vi "Get Value Variant.vi"(8 "error in (no error)":errorcluster, 10 "value":variant, 11 "value pointer in":i64) -> (0 "error out":errorcluster, 2 "value out":variant, 3 "value pointer out":i64)   [LabVIEW 2020, in "Value.lvlib"]
uses:
  Value.lvlib
  3e63842f-1b42-44b7-bfbc-53574ae558bd.vi
  94649a53-8ca4-4095-9f16-4726c07ca332.vi
  0df52538-0c37-4fc1-a2a6-aa64d23bd73e.vi
  d57c28cb-9096-4c65-b10b-a5dea6344eea.vi
  ea7cb730-9445-4e63-a674-7488b051f0a2.vi
  a983453c-48a8-483e-9635-4b6015360bbf.vi
  ecc6d044-d1d6-4258-b554-93b542f000c4.vi
  3184ba56-7df3-4453-b731-c59013ebea68.vi
  f0dd0353-13dc-4229-be36-72f5216b3ba3.vi
  6054442b-7a6b-42bc-83b9-383781339b04.vi
  663b7534-5be4-4c26-8693-775dffd107bf.vi
  6affac03-527b-4ec4-b0fc-9a513264455a.vi
  6d95b702-a3d4-47fa-b99c-6e9c691d9abd.vi
  a9131e02-a07e-4dd8-b605-98a98183cd4d.vi
  334379f0-c2c1-4fd4-b37a-a75153a3c3c1.vi
  df721e5c-d840-4c3d-88a1-754951405b27.vi
  22215a59-2fe5-468e-8a76-07a567f1422d.vi
  37bd5290-b6b7-48eb-a0fa-e2d498b26fe2.vi
  3b673ad6-c2bb-415d-ac32-dac8d0585a62.vi
  1f354738-e960-4e7d-8bfb-2b975031cf57.vi
  4907590c-51dd-452d-854a-3f23d6337043.vi
  eb45627c-0224-4171-a2ca-7d038fcf7cb5.vi
  91e94b60-106e-4a8f-bb72-5d9817169e6a.vi
  763b9c78-21ee-42ab-85a7-a612ad3e0854.vi
  c7390ac7-e1e0-4f30-b90a-9159575d946d.vi
  b475763c-3eeb-44d5-9789-6e92f77c8c05.vi
  aaf6655d-cd8e-45f8-b77e-a22837ed21e0.vi
  7e13b756-e5dd-4f30-8145-3e48ab5751a0.vi
  830d96f2-0dcb-4e12-99cb-9e6dde05f73e.vi
  311b836b-25cf-44d6-867a-da423852ab29.vi
  77dc8c9c-6059-4e17-8748-14fb7ec0ac2f.vi
  884a57a7-1cc5-4241-a283-3421418f3c32.vi
  a9875d30-4bd9-4a8c-a52c-f68dec12aa6b.vi
  e5b34253-12a8-4f36-ae48-ef8a9a19dc9f.vi
  6dbc08b8-92b8-4054-99f1-d97896c52856.vi
  9a6462e7-f1a7-4896-b94c-43e163632ccd.vi
  c55a9e90-05cb-4a8a-8098-6274f5663967.vi
  919939b4-f74b-49d6-a078-a721f5adc92b.vi
  316c9c8d-b543-4ebf-942d-59175514938d.vi
  7b5734c8-9551-4087-a43c-2e9c6be36d77.vi
  229b0493-3b28-4ef3-8240-f1556a969e00.vi
  e7c0ed72-c8d2-4a6e-8d95-57b650344be6.vi
  76e9d66a-8186-463b-a0b5-702645c41f9e.vi
  78a636ab-c8c7-43d5-9c2f-ed25fd418a22.vi
  c324c6c0-264f-44f1-9003-e2f03347ce10.vi
  3f976d8e-f489-4d6c-8102-c644feb36fb3.vi
  99229403-bf4d-41b1-8e34-2119cf99b534.vi
  2b071918-53f3-414b-a359-069b1376627a.vi
  <vilib>/Utility/error.llb/Clear Errors.vi
  <vilib>/Utility/Data Type/Get Type Information.vi
  <vilib>/Utility/Data Type/Get Array Information.vi
  <vilib>/Utility/error.llb/Error Cluster From Error Code.vi
  Get Library Path.vi
  <vilib>/ErrorRing/Error Ring.xnode
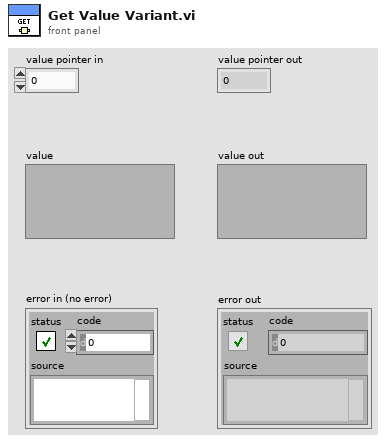
[diagram p1: front panel]
types:
  T1 = typedef "Value.lvlib/TypeCode.ctl" = enum8{"Null", "Bool", "BoolA", "Int8", "Int8A", "Int16", "Int16A", "Int32", "Int32A", "Int64", "Int64A", "UInt8", "UInt8A", "UInt16", "UInt16A", "UInt32", "UInt32A", "UInt64", "UInt64A", "Float32", "Float32A", "Float64", "Float64A", "String", "StringA", "Struct", "StructA", "Union", "UnionA", "Any", "AnyA"}
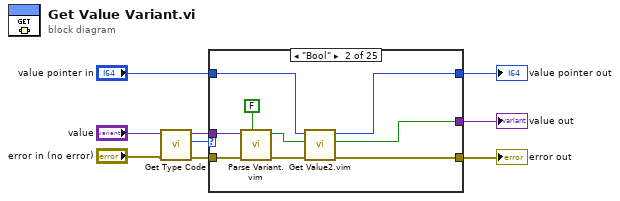
[diagram p0: block diagram]
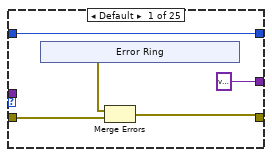
[diagram p2: hidden frame]
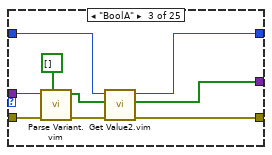
[diagram p3: hidden frame]
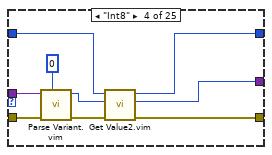
[diagram p4: hidden frame]
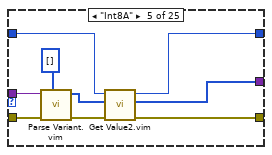
[diagram p5: hidden frame]
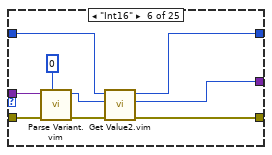
[diagram p6: hidden frame]
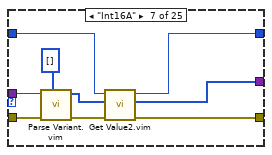
[diagram p7: hidden frame]
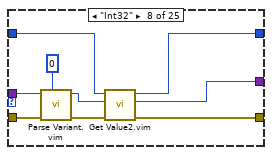
[diagram p8: hidden frame]
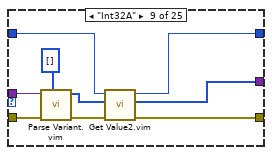
[diagram p9: hidden frame]
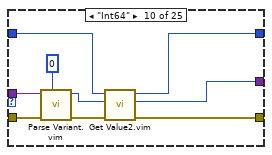
[diagram p10: hidden frame]
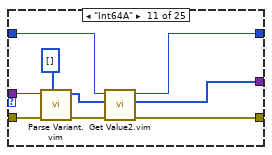
[diagram p11: hidden frame]
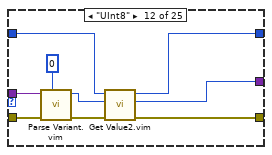
[diagram p12: hidden frame]
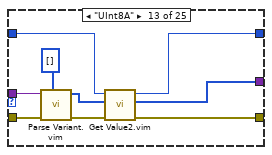
[diagram p13: hidden frame]
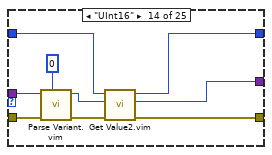
[diagram p14: hidden frame]
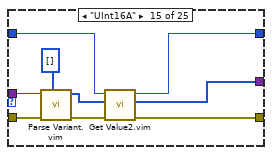
[diagram p15: hidden frame]
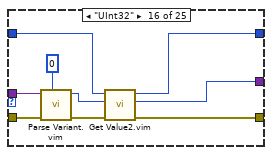
[diagram p16: hidden frame]
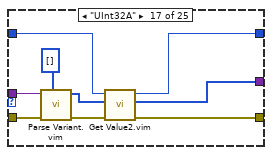
[diagram p17: hidden frame]
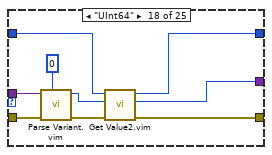
[diagram p18: hidden frame]
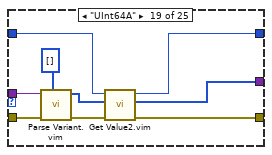
[diagram p19: hidden frame]
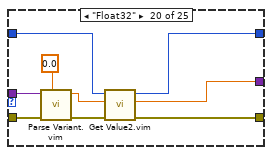
[diagram p20: hidden frame]
diagram:
  n1 = call "Get Type Code.vi"("error in (no error)"="error in (no error)", "value"="value") -> ("error out"=w7:errorcluster, "type code"=w6:T1, "value dup"=w5:variant)  [unwired: 5 in]
  n2 = case shown="\"Bool\"" w6 {
    tunnel: [w13 w24 w34 w43 w52 w61 w70 w79 w88 w97 w107 w115 w124 w133 w142 w151 w160 w169 w178 w187 w196 w205 w214 w223 w232] -> w1
    tunnel: w7 -> [w14 w27 w36 w45 w54 w63 w72 w81 w90 w99 w108 w117 w126 w135 w144 w153 w162 w171 w180 w189 w198 w207 w216 w225 w234]
    tunnel: [w10 w22 w32 w42 w50 w59 w68 w77 w86 w95 w105 w113 w122 w132 w140 w149 w159 w167 w176 w185 w194 w203 w212 w221 w230] -> w3
    tunnel: w5 -> [_ w21 w31 w41 w49 w58 w67 w76 w85 w94 w104 w112 w121 w131 w139 w148 w158 w166 w175 w184 w193 w202 w211 w220 w229]
    tunnel: [variant w20 w29 w39 w47 w56 w65 w74 w83 w92 w102 w110 w119 w129 w137 w146 w156 w164 w173 w182 w191 w200 w209 w218 w227] -> w2
    tunnel: "value pointer in" -> [w10 w19 w28 w38 w46 w55 w64 w73 w82 w91 w100 w109 w118 w128 w136 w145 w155 w163 w172 w181 w190 w199 w208 w217 w226]
    frame Default {
      n3 = xnode "Error Ring"() -> ("error out"=w12:errorcluster)
      n4 = Merge Errors(w12, w14) -> (w13:errorcluster)
    }
    frame "Bool" {
      n5 = call "Parse Variant.vim"("default"=FALSE, "error in (no error)"=w27, "value"=w21) -> ("error out"=w25:errorcluster, "value out"=w23:bool)  [unwired: 7 in]
      n6 = call "Get Value2.vim"("error in"=w25, "default"=w23, "value pointer in"=w19) -> ("error out"=w24:errorcluster, "value"=w20:bool, "value pointer out"=w22:i64)  [unwired: 6 in]
    }
    frame "BoolA" {
      n7 = call "Parse Variant.vim"("default"=bool[] [], "error in (no error)"=w36, "value"=w31) -> ("error out"=w35:errorcluster, "value out"=w33:bool[])  [unwired: 7 in]
      n8 = call "Get Value2.vim"("error in"=w35, "default"=w33, "value pointer in"=w28) -> ("error out"=w34:errorcluster, "value"=w29:bool[], "value pointer out"=w32:i64)  [unwired: 6 in]
    }
    frame "Int8" {
      n9 = call "Parse Variant.vim"("default"=i8 0, "error in (no error)"=w45, "value"=w41) -> ("error out"=w44:errorcluster, "value out"=w37:i8)  [unwired: 7 in]
      n10 = call "Get Value2.vim"("error in"=w44, "default"=w37, "value pointer in"=w38) -> ("error out"=w43:errorcluster, "value"=w39:i8, "value pointer out"=w42:i64)  [unwired: 6 in]
    }
    frame "Int8A" {
      n11 = call "Parse Variant.vim"("default"=i8[] [], "error in (no error)"=w54, "value"=w49) -> ("error out"=w53:errorcluster, "value out"=w51:i8[])  [unwired: 7 in]
      n12 = call "Get Value2.vim"("error in"=w53, "default"=w51, "value pointer in"=w46) -> ("error out"=w52:errorcluster, "value"=w47:i8[], "value pointer out"=w50:i64)  [unwired: 6 in]
    }
    frame "Int16" {
      n13 = call "Parse Variant.vim"("default"=i16 0, "error in (no error)"=w63, "value"=w58) -> ("error out"=w62:errorcluster, "value out"=w60:i16)  [unwired: 7 in]
      n14 = call "Get Value2.vim"("error in"=w62, "default"=w60, "value pointer in"=w55) -> ("error out"=w61:errorcluster, "value"=w56:i16, "value pointer out"=w59:i64)  [unwired: 6 in]
    }
    frame "Int16A" {
      n15 = call "Parse Variant.vim"("default"=i16[] [], "error in (no error)"=w72, "value"=w67) -> ("error out"=w71:errorcluster, "value out"=w69:i16[])  [unwired: 7 in]
      n16 = call "Get Value2.vim"("error in"=w71, "default"=w69, "value pointer in"=w64) -> ("error out"=w70:errorcluster, "value"=w65:i16[], "value pointer out"=w68:i64)  [unwired: 6 in]
    }
    frame "Int32" {
      n17 = call "Parse Variant.vim"("default"=0, "error in (no error)"=w81, "value"=w76) -> ("error out"=w80:errorcluster, "value out"=w78:i32)  [unwired: 7 in]
      n18 = call "Get Value2.vim"("error in"=w80, "default"=w78, "value pointer in"=w73) -> ("error out"=w79:errorcluster, "value"=w74:i32, "value pointer out"=w77:i64)  [unwired: 6 in]
    }
    frame "Int32A" {
      n19 = call "Parse Variant.vim"("default"=i32[] [], "error in (no error)"=w90, "value"=w85) -> ("error out"=w89:errorcluster, "value out"=w87:i32[])  [unwired: 7 in]
      n20 = call "Get Value2.vim"("error in"=w89, "default"=w87, "value pointer in"=w82) -> ("error out"=w88:errorcluster, "value"=w83:i32[], "value pointer out"=w86:i64)  [unwired: 6 in]
    }
    frame "Int64" {
      n21 = call "Parse Variant.vim"("default"=i64 0, "error in (no error)"=w99, "value"=w94) -> ("error out"=w98:errorcluster, "value out"=w96:i64)  [unwired: 7 in]
      n22 = call "Get Value2.vim"("error in"=w98, "default"=w96, "value pointer in"=w91) -> ("error out"=w97:errorcluster, "value"=w92:i64, "value pointer out"=w95:i64)  [unwired: 6 in]
    }
    frame "Int64A" {
      n23 = call "Parse Variant.vim"("default"=i64[] [], "error in (no error)"=w108, "value"=w104) -> ("error out"=w101:errorcluster, "value out"=w106:i64[])  [unwired: 7 in]
      n24 = call "Get Value2.vim"("error in"=w101, "default"=w106, "value pointer in"=w100) -> ("error out"=w107:errorcluster, "value"=w102:i64[], "value pointer out"=w105:i64)  [unwired: 6 in]
    }
    frame "UInt8" {
      n25 = call "Parse Variant.vim"("default"=u8 0, "error in (no error)"=w117, "value"=w112) -> ("error out"=w116:errorcluster, "value out"=w114:u8)  [unwired: 7 in]
      n26 = call "Get Value2.vim"("error in"=w116, "default"=w114, "value pointer in"=w109) -> ("error out"=w115:errorcluster, "value"=w110:u8, "value pointer out"=w113:i64)  [unwired: 6 in]
    }
    frame "UInt8A" {
      n27 = call "Parse Variant.vim"("default"=u8[] [], "error in (no error)"=w126, "value"=w121) -> ("error out"=w125:errorcluster, "value out"=w123:u8[])  [unwired: 7 in]
      n28 = call "Get Value2.vim"("error in"=w125, "default"=w123, "value pointer in"=w118) -> ("error out"=w124:errorcluster, "value"=w119:u8[], "value pointer out"=w122:i64)  [unwired: 6 in]
    }
    frame "UInt16" {
      n29 = call "Parse Variant.vim"("default"=u16 0, "error in (no error)"=w135, "value"=w131) -> ("error out"=w134:errorcluster, "value out"=w127:u16)  [unwired: 7 in]
      n30 = call "Get Value2.vim"("error in"=w134, "default"=w127, "value pointer in"=w128) -> ("error out"=w133:errorcluster, "value"=w129:u16, "value pointer out"=w132:i64)  [unwired: 6 in]
    }
    frame "UInt16A" {
      n31 = call "Parse Variant.vim"("default"=u16[] [], "error in (no error)"=w144, "value"=w139) -> ("error out"=w143:errorcluster, "value out"=w141:u16[])  [unwired: 7 in]
      n32 = call "Get Value2.vim"("error in"=w143, "default"=w141, "value pointer in"=w136) -> ("error out"=w142:errorcluster, "value"=w137:u16[], "value pointer out"=w140:i64)  [unwired: 6 in]
    }
    frame "UInt32" {
      n33 = call "Parse Variant.vim"("default"=u32 0, "error in (no error)"=w153, "value"=w148) -> ("error out"=w152:errorcluster, "value out"=w150:u32)  [unwired: 7 in]
      n34 = call "Get Value2.vim"("error in"=w152, "default"=w150, "value pointer in"=w145) -> ("error out"=w151:errorcluster, "value"=w146:u32, "value pointer out"=w149:i64)  [unwired: 6 in]
    }
    frame "UInt32A" {
      n35 = call "Parse Variant.vim"("default"=u32[] [], "error in (no error)"=w162, "value"=w158) -> ("error out"=w161:errorcluster, "value out"=w154:u32[])  [unwired: 7 in]
      n36 = call "Get Value2.vim"("error in"=w161, "default"=w154, "value pointer in"=w155) -> ("error out"=w160:errorcluster, "value"=w156:u32[], "value pointer out"=w159:i64)  [unwired: 6 in]
    }
    frame "UInt64" {
      n37 = call "Parse Variant.vim"("default"=u64 0, "error in (no error)"=w171, "value"=w166) -> ("error out"=w170:errorcluster, "value out"=w168:u64)  [unwired: 7 in]
      n38 = call "Get Value2.vim"("error in"=w170, "default"=w168, "value pointer in"=w163) -> ("error out"=w169:errorcluster, "value"=w164:u64, "value pointer out"=w167:i64)  [unwired: 6 in]
    }
    frame "UInt64A" {
      n39 = call "Parse Variant.vim"("default"=u64[] [], "error in (no error)"=w180, "value"=w175) -> ("error out"=w179:errorcluster, "value out"=w177:u64[])  [unwired: 7 in]
      n40 = call "Get Value2.vim"("error in"=w179, "default"=w177, "value pointer in"=w172) -> ("error out"=w178:errorcluster, "value"=w173:u64[], "value pointer out"=w176:i64)  [unwired: 6 in]
    }
    frame "Float32" {
      n41 = call "Parse Variant.vim"("default"=sgl 0.0, "error in (no error)"=w189, "value"=w184) -> ("error out"=w188:errorcluster, "value out"=w186:sgl)  [unwired: 7 in]
      n42 = call "Get Value2.vim"("error in"=w188, "default"=w186, "value pointer in"=w181) -> ("error out"=w187:errorcluster, "value"=w182:sgl, "value pointer out"=w185:i64)  [unwired: 6 in]
    }
    frame "Float64" {
      n43 = call "Parse Variant.vim"("default"=0.0, "error in (no error)"=w198, "value"=w193) -> ("error out"=w197:errorcluster, "value out"=w195:dbl)  [unwired: 7 in]
      n44 = call "Get Value2.vim"("error in"=w197, "default"=w195, "value pointer in"=w190) -> ("error out"=w196:errorcluster, "value"=w191:dbl, "value pointer out"=w194:i64)  [unwired: 6 in]
    }
    frame "Float32A" {
      n45 = call "Parse Variant.vim"("default"=sgl[] [], "error in (no error)"=w207, "value"=w202) -> ("error out"=w206:errorcluster, "value out"=w204:sgl[])  [unwired: 7 in]
      n46 = call "Get Value2.vim"("error in"=w206, "default"=w204, "value pointer in"=w199) -> ("error out"=w205:errorcluster, "value"=w200:sgl[], "value pointer out"=w203:i64)  [unwired: 6 in]
    }
    frame "Float64A" {
      n47 = call "Parse Variant.vim"("default"=dbl[] [], "error in (no error)"=w216, "value"=w211) -> ("error out"=w215:errorcluster, "value out"=w213:dbl[])  [unwired: 7 in]
      n48 = call "Get Value2.vim"("error in"=w215, "default"=w213, "value pointer in"=w208) -> ("error out"=w214:errorcluster, "value"=w209:dbl[], "value pointer out"=w212:i64)  [unwired: 6 in]
    }
    frame "String" {
      n49 = call "Parse Variant.vim"("default"="", "error in (no error)"=w225, "value"=w220) -> ("error out"=w224:errorcluster, "value out"=w222:string)  [unwired: 7 in]
      n50 = call "Get Value2.vim"("error in"=w224, "default"=w222, "value pointer in"=w217) -> ("error out"=w223:errorcluster, "value"=w218:string, "value pointer out"=w221:i64)  [unwired: 6 in]
    }
    frame "StringA" {
      n51 = call "Parse Variant.vim"("default"=string[] [], "error in (no error)"=w234, "value"=w229) -> ("error out"=w233:errorcluster, "value out"=w231:string[])  [unwired: 7 in]
      n52 = call "Get Value2.vim"("error in"=w233, "default"=w231, "value pointer in"=w226) -> ("error out"=w232:errorcluster, "value"=w227:string[], "value pointer out"=w230:i64)  [unwired: 6 in]
    }
  }
  "value pointer out" <- w3
  "value out" <- w2
  "error out" <- w1
